vi "DigitalWrite.vi"(2 "error in (no error)":errorcluster, 3 "DOdata":bool[](array[boolean]), 4 "DOpins":i32[](array[numeric]), 5 "InputData":cluster{"String":string, "userdata":string}) -> (0 "error out":errorcluster, 1 "OutputData":cluster{"String":string, string})   [LabVIEW 2017]
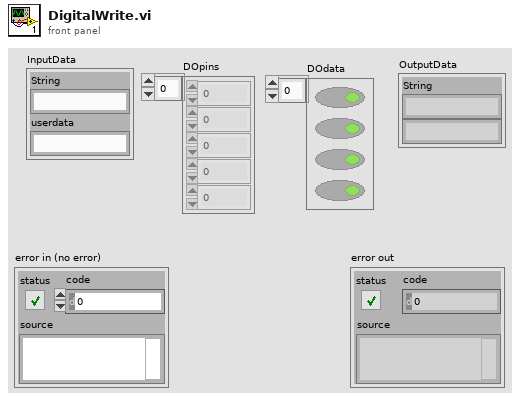
[diagram p1: front panel]
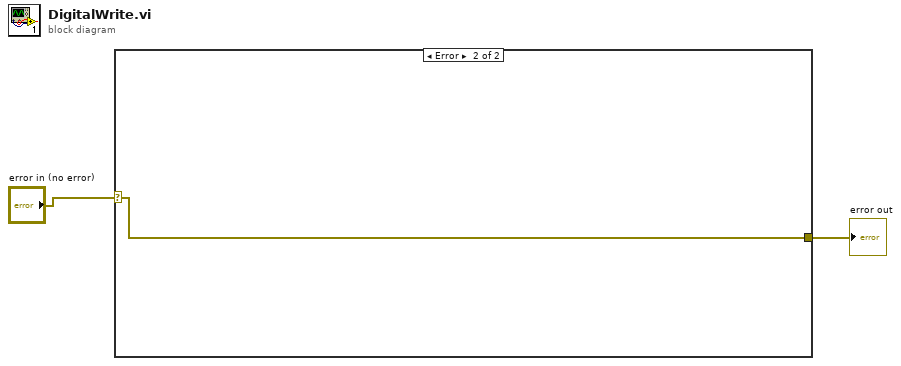
[diagram p0: block diagram]
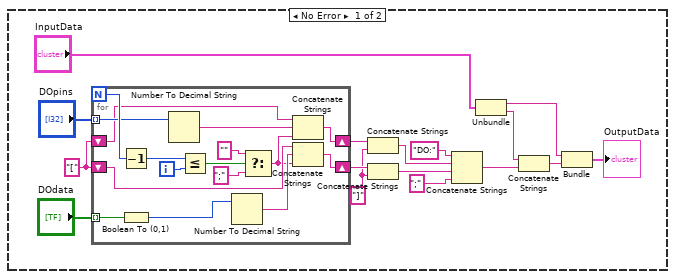
[diagram p2: hidden frame]
diagram:
  n1 = case shown="Error" "error in (no error)" {
    selector: "error in (no error)" -> [_ w35]
    tunnel: [_ w35] -> w1
    frame No Error {
      w10 = "]"
      w13 = "["
      n2 = for {
        N -> [w34]
        shift-right: [w25] -> w17
        shift-left: w13 -> [w28]
        tunnel: "DOpins" -> [w24] mode=indexing
        shift-right: [w20] -> w11
        shift-left: w13 -> [w22]
        tunnel: "DOdata" -> [w19] mode=indexing
        i -> [w33]
        n3 = Decrement(x=w34) -> (x-1=w29:i32)
        n4 = Boolean To (0,1)(Boolean=w19) -> (0, 1=w27:i16)
        n5 = Number To Decimal String(number=w24) -> (decimal integer string=w23:string)  [unwired: 1 in]
        n6 = Less Or Equal?(x=w29, y=w33) -> (x <= y?=w32:bool)
        n7 = Number To Decimal String(number=w27) -> (decimal integer string=w26:string)  [unwired: 1 in]
        n8 = Select(t="" ("string"), s=w32, f=";" ("string")) -> (s? t:f=w21:string)
        n9 = Concatenate Strings(w22, w23, w21) -> (w20:string)
        n10 = Concatenate Strings(w28, w26, w21) -> (w25:string)
      }
      n11 = Concatenate Strings(w11, w10) -> (w9:string)
      n12 = Concatenate Strings(w17, w10) -> (w18:string)
      n13 = Concatenate Strings("DO:" ("url"), w9, w18, ";") -> (w8:string)
      n14 = Unbundle("InputData") -> ("String"=w5:string, "userdata"=w7:string)
      n15 = Concatenate Strings(w7, w8) -> (w4:string)
      n16 = Bundle("String"=w5, w4) -> (→"OutputData":cluster{"String":string, string})  [unwired: 1 in]
    }
    frame Error {
    }
  }
  "error out" <- w1
